vi "Data from Channel 1.vi"() -> (3 "Channels Data":i16[](array[numeric]))   [LabVIEW 2012]
uses:
  <vilib>/rvi/eio/common/nirviEmuTemplateMethod_errors.vi
  <vilib>/eio/EIONode/EIONode.xnode
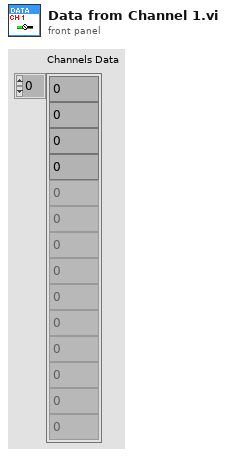
[diagram p1: front panel]
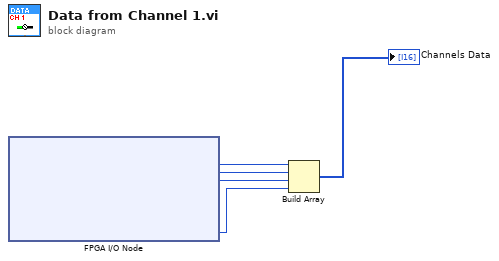
[diagram p0: block diagram]
diagram:
  n1 = xnode "FPGA I/O Node"() -> ("IO Module\\AI 1 Data N-3"=w5:i16, "IO Module\\AI 1 Data N-2"=w4:i16, "IO Module\\AI 1 Data N-1"=w3:i16, "IO Module\\AI 1 Data N"=w2:i16)  [unwired: 4 in, 4 out]
  n2 = Build Array(w5, w4, w3, w2) -> (→"Channels Data":i16[])
